vi "EnabledStatusChanged.vi"(8 "error in (no error)":errorcluster, 10 "GISHeadStatus":T1[](array[typedef]), 11 "GISHeadStatus Old":T1[](array[typedef])) -> (0 "error out":errorcluster, 3 "State":string)   [LabVIEW 2022 SP3, in "TopLevel.lvclass"]
uses:
  TopLevel.lvclass
  GIS Printer/Typedefs/GIS Status--Cluster.ctl
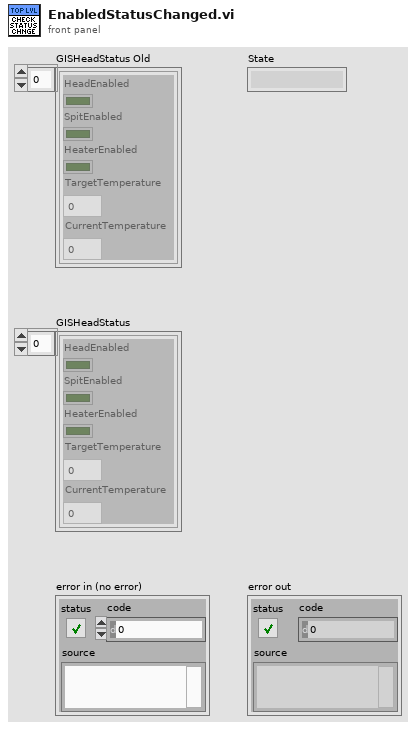
[diagram p1: front panel]
types:
  T1 = typedef "GIS Status--Cluster.ctl" = cluster{"HeadEnabled":bool, "SpitEnabled":bool, "HeaterEnabled":bool, "TargetTemperature":dbl, "CurrentTemperature":dbl}
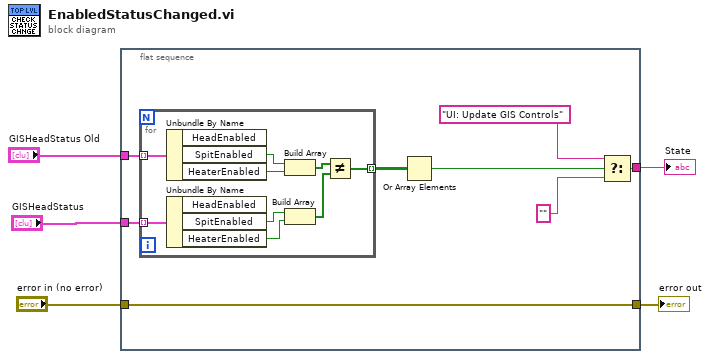
[diagram p0: block diagram]
diagram:
  n1 = flat-sequence {
    tunnel: "GISHeadStatus Old" -> [w12]
    tunnel: "GISHeadStatus" -> [w11]
    tunnel: [w6] -> w3
    tunnel: "error in (no error)" -> [w13]
    tunnel: [w13] -> w5
    frame #0 {
      n2 = for {
        tunnel: w12 -> [w22] mode=indexing
        tunnel: w11 -> [w21] mode=indexing
        tunnel: [w14] -> w10 mode=indexing
        n3 = Unbundle By Name(w22) -> ("SpitEnabled"=w20:bool, "HeaterEnabled"=w19:bool)  [unwired: 1 out]
        n4 = Unbundle By Name(w21) -> ("SpitEnabled"=w18:bool, "HeaterEnabled"=w17:bool)  [unwired: 1 out]
        n5 = Build Array(w20, w19) -> (w16:bool[])
        n6 = Build Array(w18, w17) -> (w15:bool[])
        n7 = Not Equal?(x=w16, y=w15) -> (x != y?=w14:bool[])
      }
      n8 = Or Array Elements(Boolean array=w10) -> (logical OR=w9:bool)
      n9 = Select(t="UI: Update GIS Controls", s=w9, f="") -> (s? t:f=w6:string)
    }
  }
  "error out" <- w5
  "State" <- w3
